vi "DAQ.vi"() -> ()   [LabVIEW 2018]
uses:
  <vilib>/userdefined/High Color/nirio_resource_hc.ctl
  Turbo Instrument Controller.llb/Type Def - Gauge Num Selection.ctl
  <vilib>/Utility/file.llb/Read Delimited Spreadsheet (DBL).vi
  <vilib>/FPGAPlugInAG/PXIe-7856R/niLvFpga_Open_PXIe-7856R.vi
  <vilib>/rvi/interface/nirviOpenFPGA/nirviOpenFPGA.xnode
  FPGA code/FPGA Bitfiles/Microspherefeedb_FPGATarget2_MultiChannelfFee_SMENcAWM-fA.lvbitx
  <instrlib>/Agilent 2000 3000 X-Series/Agilent 2000 3000 X-Series.lvlib
panel:
  in  "Synth_sync":bool
  in  "Scope only?":bool=TRUE
  in  "RIO Device":T1="RIO0"
  out "error out":errorcluster
  in  "Range (S)":dbl=0.002 format="%#_13g"
  in  "Use osciloscope chan 1":bool=TRUE
  in  "use single channel":bool
  in  "EOM":T2={"QWP"=FALSE, "QWP angles"="125,124,123,122,121,120,119,118,117,116,115,114,113,112,111,110,109,108,107,106,105,104,103,102,101,100,99,98,97,96,95,94,93,92,91,90,89,88,87,86,85,84,83,82,81,80,79,78,77,76,75,74,73,72,71,70,69,68,67,66,65,64,63,62,61,60,59,58,57,56,55,54,53,52,51,50,49,48,47,46,45,44,43,42,41,40,39,38,37,36,35,34,33,32,31,30,29,28,27,26,25,24,23,22,21", "reverse"=FALSE}
  out "Axes position":i32[](array[numeric])
  in  "Arb waveform path":path=path "C:/Users/UsphereLab/Documents/GitHub/Optlev/scripts/freq_comb/freq_comb_fixed4.txt"
  in  "Dipole average settings":T3={"Initial wait time"=5.0, "Number of steps"=10000, "CH1 Voltage"=13.5, "Use?"=FALSE, "CH2 Voltage"=13.5, "Variable Steps"=FALSE}
  in  "Stage settings":T4={"thetaY steps"=-12.0, "thetaZ steps"=-20.0, "Run thetaY?"=FALSE, "Run thetaZ?"=FALSE, "# repeats \n   in thetaY"=1, "# repeats \n   in thetaZ"=100}
  in  "Trigger Synth":bool
  in  "Enable Output?":bool
  out "P_cc [torr]":dbl format="%#_3g"
  out "P_pirani [torr]":dbl format="%#_3g"
  out "T_elec_rack [C]":dbl
  out "T_opt_table [C]":dbl
  in  "Read pressures?":bool
  in  "Flash lamp\n settings:":T5={"Flash lamp?"=FALSE, "Number of cyles\nbetween flashes"=1, "# Pulses"=1, "Stop flashing \nbelow thresh?"=FALSE, "Stop threshold"=0.02, "Pulse amp (V)"=0.001}
  in  "Synth settings:":T6={"start volt (V)"=0.0, "stop volt (V) "=0.0, "# V Steps"=1, "start freq (Hz)"=48.0, "stop freq (Hz) "=48.0, "# F steps"=1, "dc offset?"=FALSE, "start DC (V)"=0.0, "stop DC (V)"=0.0, "# DC steps "=1, "Set synth\n(HP33120A)?"=FALSE, "Use arbitrary\nwaveform?"=FALSE, "Arb waveform name:"="VOLATILE"}
  out "Waveform \nGraph":dbl[][](graph)
  out "Curr threshold":dbl
  in  "Number of Samples":dbl=100000.0
  in  "Sample Rate [Hz]":dbl=10000.0
  out "Actual Sample \nRate":dbl=10000.0 format="%0.2f"
  in  "Delay between files [s]":dbl caption="Delay Time (s)"
  in  "Num files":i32=1
  in  "File base name":string="rot9"
  in  "Directory path":path=path "C:/data/GADI"
  # "Logging Settings"
  # "How to use the channel/scope statements:\n\n\"use single channel\":\n\nis for measurement of rotation using the daq\nand high sample rate\n\n\n\n\"Scope only\" and  \"Use osciloscope chan 1\":\n\nonly uses the channel 1 of the scope\n\n\n\n \"Use osciloscope chan 1\":\n\nuses daq together with the channel 1 of the scope\n\nWarning: for this option to work, the number of samples per daq channel must be the same of the scope: ie; NS = 50e4"
  # "524288"
  # "Environment"
  # "Starts with the positive voltage\n\nIf Variable Steps is on, then the voltages in the synth's AC input and the voltages for the dipole will change for each step by 10% of the original voltage, so that we have voltages\n1*V volts, 0.9*V volts, 0.8*V volts, 0.7*V volts, and back again to V volts"
  # "Flash Lamp Settings"
  # "Acquired Data"
  # "Timing Settings"
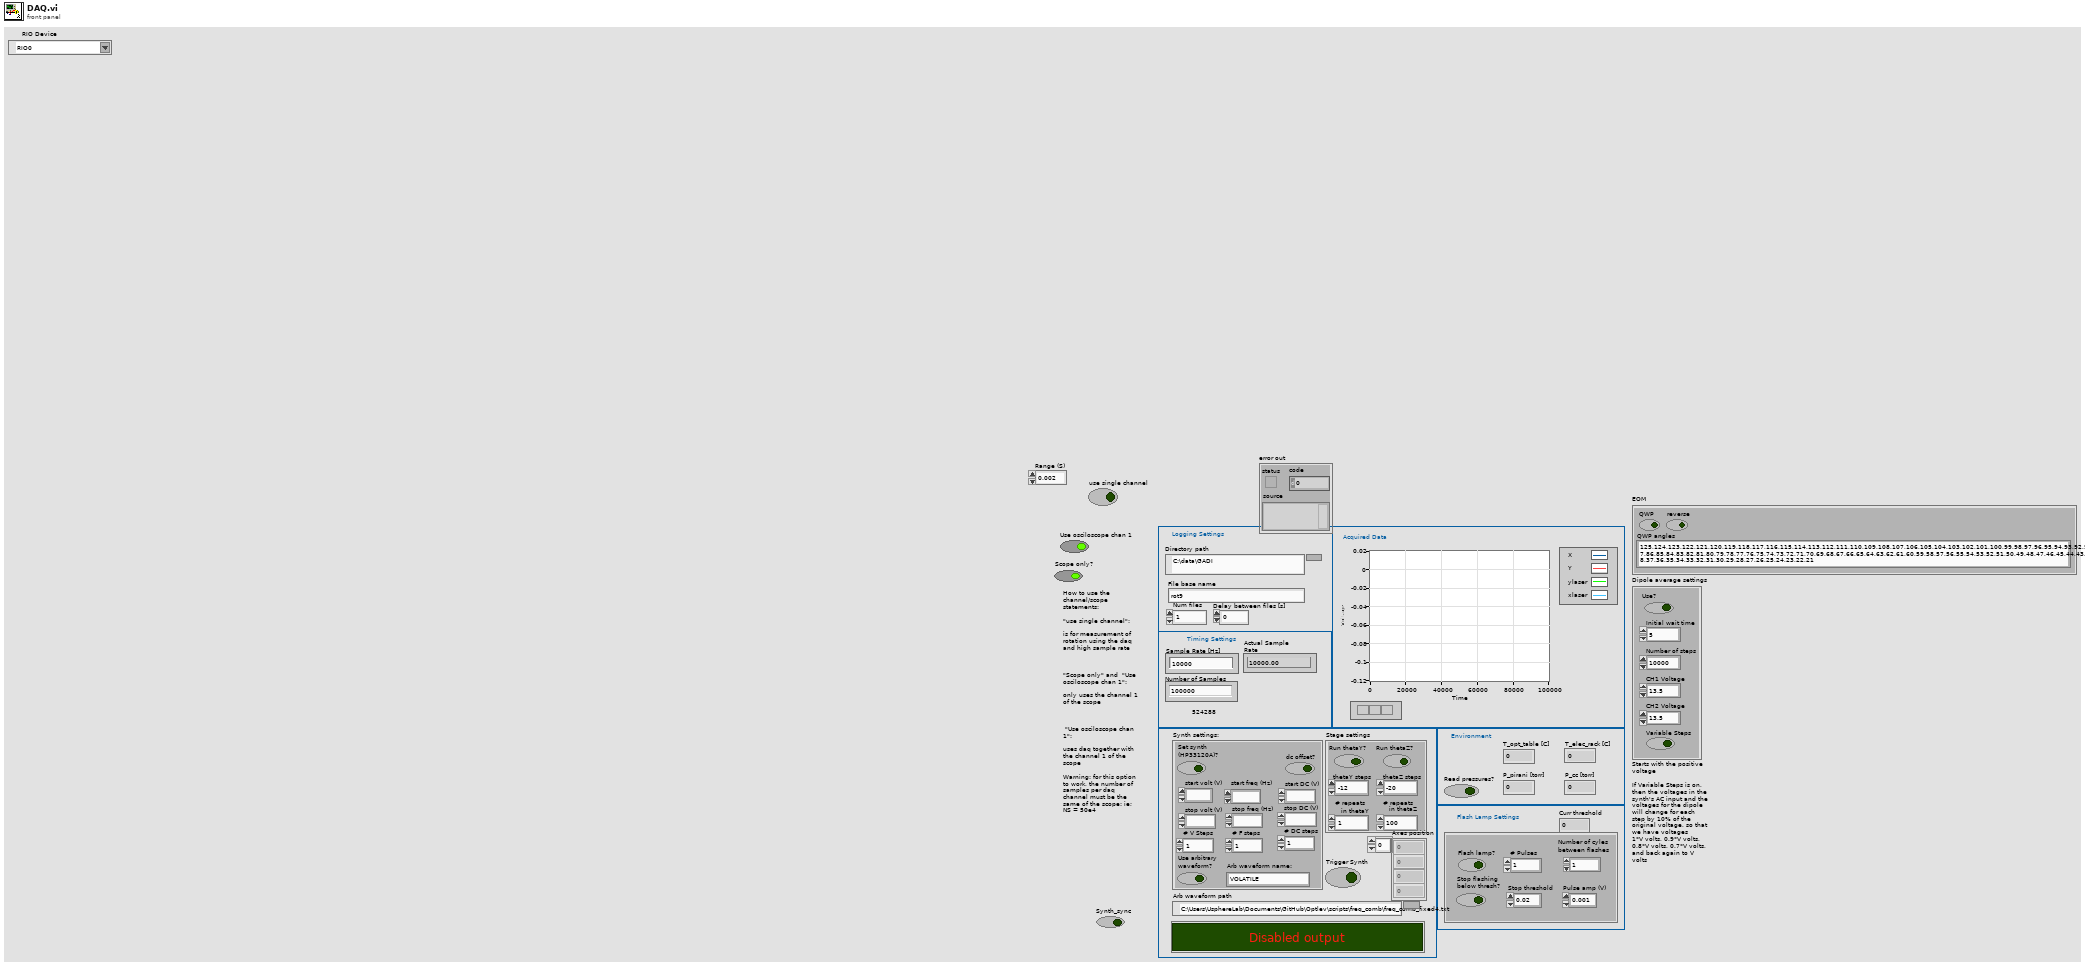
[diagram p1: front panel]
types:
  T1 = typedef "nirio_resource_hc.ctl" = tag
  T2 = cluster{"QWP":bool, "QWP angles":string, "reverse":bool}
  T3 = cluster{"Initial wait time":dbl, "Number of steps":i32, "CH1 Voltage":dbl, "Use?":bool, "CH2 Voltage":dbl, "Variable Steps":bool}
  T4 = cluster{"thetaY steps":dbl, "thetaZ steps":dbl, "Run thetaY?":bool, "Run thetaZ?":bool, "# repeats \n   in thetaY":i32, "# repeats \n   in thetaZ":i32}
  T5 = cluster{"Flash lamp?":bool, "Number of cyles\nbetween flashes":i32, "# Pulses":i32, "Stop flashing \nbelow thresh?":bool, "Stop threshold":dbl, "Pulse amp (V)":dbl}
  T6 = cluster{"start volt (V)":ext, "stop volt (V) ":ext, "# V Steps":i32, "start freq (Hz)":ext, "stop freq (Hz) ":ext, "# F steps":i32, "dc offset?":bool, "start DC (V)":ext, "stop DC (V)":ext, "# DC steps ":i32, "Set synth\n(HP33120A)?":bool, "Use arbitrary\nwaveform?":bool, "Arb waveform name:":string}
  T7 = cluster{"Tot Synth Arr":dbl[], "Tot Stage Arr":dbl[], "Stage Name Arr":dbl[], "QWP":dbl}[]
  T8 = cluster{"synth cluster":cluster{"VISA resource name out":refnum<visa-resource-name>, "error out":errorcluster}, "tilt stage config":cluster{"Y error out":errorcluster, "Y CmdLib Out":refnum<k24>, "Y Device Address":i32, "Y DeviceKey Out":string, "Z error out":errorcluster, "Z CmdLib Out":refnum<k24>, "Z Device Address":i32, "Z DeviceKey Out":string}}
  T9 = cluster{"Number of Samples":dbl, "Sample Rate [Hz]":dbl, "Physical Channels (Position signals)":tag, "Sample Clock Source":tag}
  T10 = typedef "Type Def - Gauge Num Selection.ctl" = enum16{"Gauge 1", "Gauge 2", "Gauge 3", "Gauge 4", "Gauge 5", "Gauge 6"}
  T11 = cluster{"Tot Synth Arr":dbl[], "Tot Stage Arr":dbl[], "Stage Name Arr":dbl[], "QWP":dbl}
  T12 = cluster{"Output channel (for flashing)":tag, i32, "path out":path, "Flash lamp\n settings:":cluster{"Flash lamp?":bool, "Number of cyles\nbetween flashes":i32, "# Pulses":i32, "Stop flashing \nbelow thresh?":bool, "Stop threshold":dbl, "Pulse amp (V)":dbl}}
  T13 = cluster{"Use arbitrary\nwaveform?":bool, "Arb waveform name:":string, "Enable Output?":bool, "Trigger Synth":bool, i32, "first row":dbl[]}
  T14 = cluster{"VISA resource name out":refnum<visa-resource-name>, "error out":errorcluster}
  T15 = cluster{"task out":refnum<k21>, "error out":errorcluster, "SampClk.Rate":dbl}
  T16 = cluster{"task out":refnum<k21>, "error out":errorcluster}
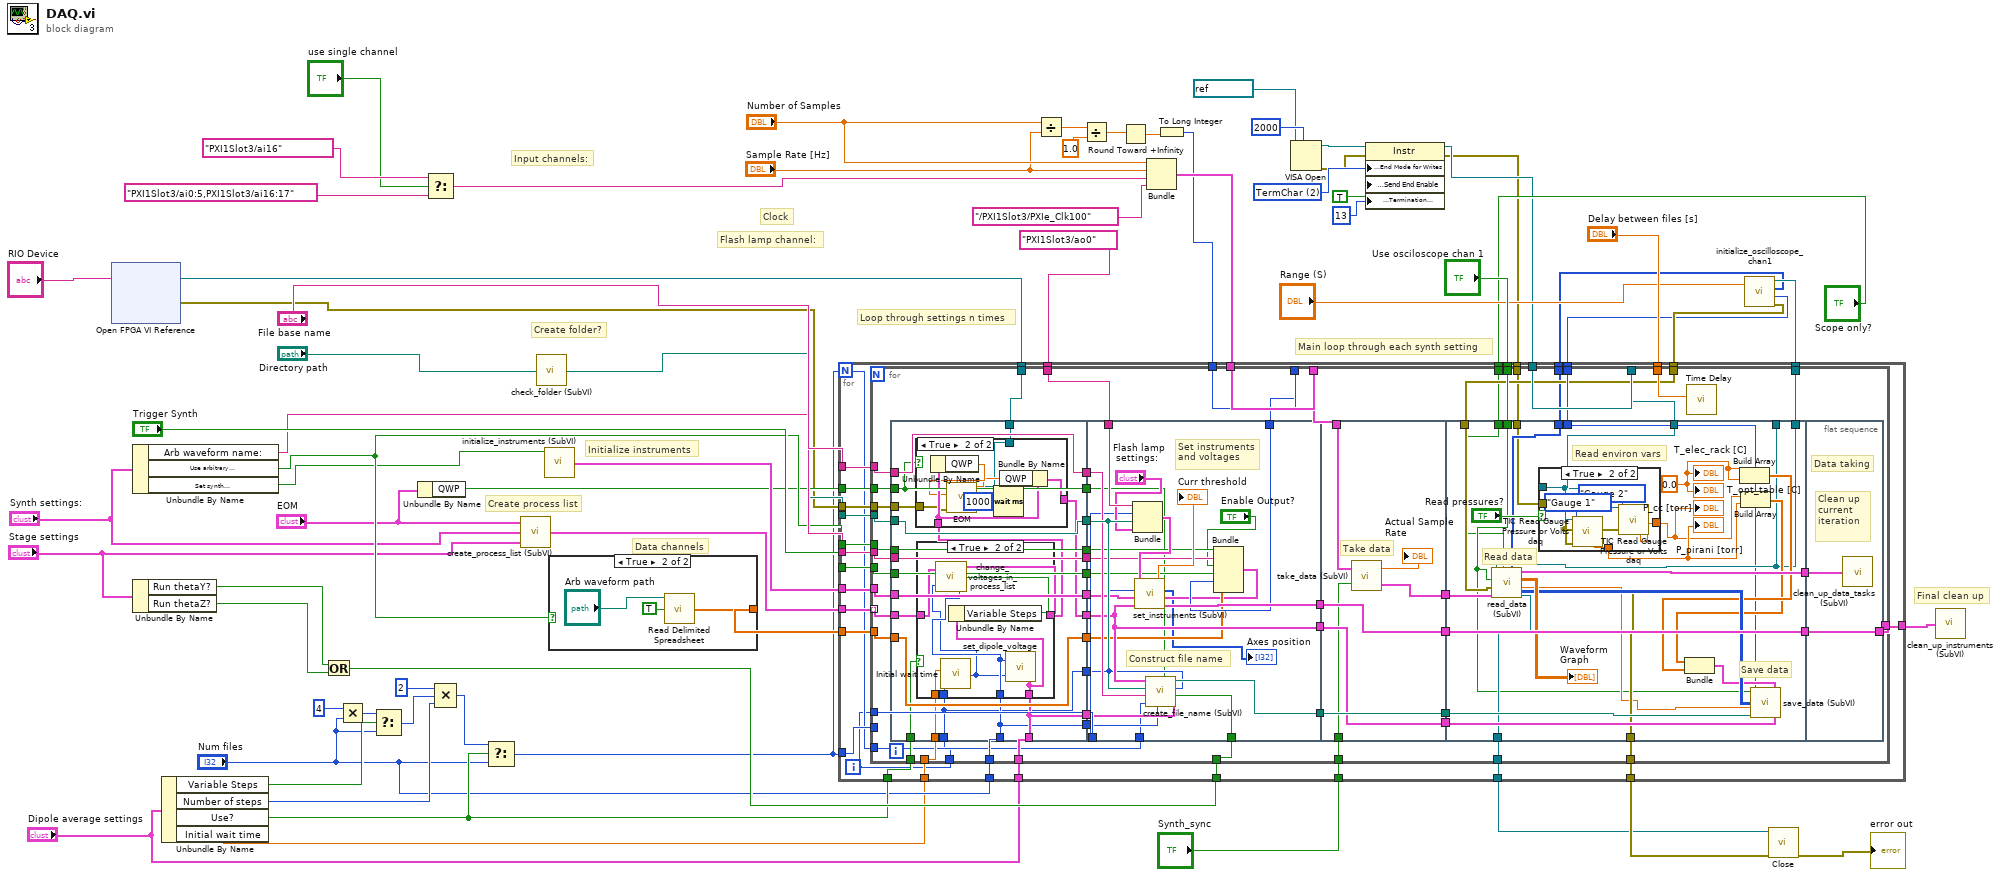
[diagram p0: block diagram]
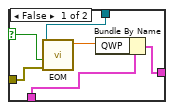
[diagram p2: hidden frame]
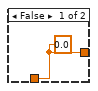
[diagram p4: hidden frame]
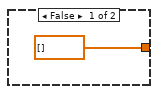
[diagram p5: hidden frame]
diagram:
  w8 = u16 2 items=["None", "Last Bit", "TermChar", "Break"] ("Serial Settings:End Mode for Writes")
  # "Main loop through each synth setting"
  # "Loop through settings n times"
  # "Final clean up"
  # "Initialize instruments"
  # "Create process list"
  # "Create folder?"
  # "Clock"
  # "Data channels"
  # "Flash lamp channel:"
  # "Input channels:"
  n1 = xnode "Open FPGA VI Reference"("resource name"="RIO Device") -> ("FPGA VI Reference Out"=w11:refnum<k20>, "error out"=w14:errorcluster)  [unwired: 1 in]
  n2 = Unbundle By Name("Synth settings:") -> ("Arb waveform name:"=w59:string, "Use arbitrary\nwaveform?"=w50:bool, "Set synth\n(HP33120A)?"=w43:bool)
  n3 = Unbundle By Name("Stage settings") -> ("Run thetaY?"=w48:bool, "Run thetaZ?"=w49:bool)
  n4 = Unbundle By Name("Dipole average settings") -> ("Variable Steps"=w37:bool, "Number of steps"=w41:i32, "Use?"=w38:bool, "Initial wait time"=w32:dbl)
  n5 = Or(x=w48, y=w49) -> (x .or. y?=w45:bool)
  n6 = Multiply(x=4, y="Num files") -> (x*y=w36:i32)
  n7 = Select(t=w36, s=w37, f="Num files") -> (s? t:f=w34:i32)
  n8 = Unbundle By Name("EOM") -> ("QWP"=w30:bool)
  n9 = Select(t=tag "PXI1Slot3/ai16" ("Physical Channels (Position signals)"), s="use single channel", f=tag "PXI1Slot3/ai0:5,PXI1Slot3/ai16:17" ("Physical Channels (Position signals)")) -> (s? t:f=w27:tag)
  n10 = Compound Arithmetic op=MULTIPLY(2 ("value"), w34, w41) -> (w40:i32)
  n11 = Select(t=w40, s=w38, f="Num files") -> (s? t:f=w12:i32)
  n12 = call "create_process_list (SubVI).vi"("Stage settings"="Stage settings", "Synth settings:"="Synth settings:", "Quarter Wave Plate"="EOM") -> ("Process list"=w55:T7)
  n13 = call "check_folder (SubVI).vi"("path in"="Directory path") -> ("path out"=w54:path)
  n14 = call "initialize_instruments (SubVI).vi"("Use synth?"=w43) -> ("initialized output"=w53:T8)  [unwired: 2 in]
  n15 = case shown="True" w50 {
    tunnel: [dbl[] [] ("first row") w72] -> w52
    frame False {
    }
    frame True {
      n16 = call-poly <vilib>:"Read Delimited Spreadsheet.vi"("file path (dialog if empty)"="Arb waveform path", "transpose? (F)"=TRUE) -> ("first row"=w72:dbl[])  [unwired: 8 in, 5 out]
    }
  }
  n17 = Divide(x="Number of Samples", y="Sample Rate [Hz]") -> (x/y=w63:dbl)
  n18 = Divide(x=w63, y=1.0) -> (x/y=w57:dbl)
  n19 = Round Toward +Infinity(x=w57) -> (ceil(x): smallest int >= x=w56:dbl)
  n20 = Bundle("Number of Samples"="Number of Samples", "Sample Rate [Hz]"="Sample Rate [Hz]", "Physical Channels (Position signals)"=w27, "Sample Clock Source"=tag "/PXI1Slot3/PXIe_Clk100") -> (w67:T9)  [unwired: 1 in]
  n21 = To Long Integer(number=w56) -> (32bit integer=w60:i32)
  n22 = VISA Open(timeout (0)=u32 2000 ("VISA Open timeout (0)"), VISA resource name=refnum<visa-resource-name> "COM7") -> (VISA resource name=w5:refnum<visa-resource-name>, error out=w4:errorcluster)  [unwired: 3 in]
  n23 = property class="Instr"(reference=w5, error in=w4, "Serial Settings:End Mode for Writes"=w8, "Message Based Settings:Send End Enable"=TRUE, "Message Based Settings:Termination Character"=u8 13) -> (reference out=w3:refnum<visa-resource-name>, error out=w1:errorcluster)
  n24 = call "initialize_oscilloscope_chan1.vi"("Range (0.001 S)"="Range (S)") -> ("VISA resource name out"=w18:refnum<visa-resource-name>, "channels"=w17:i32[], "number"=w16:i32, "error out"=w19:errorcluster)  [unwired: 1 in]
  n25 = for {
    N: w12 -> [w76]
    tunnel: w55 -> [w107]
    tunnel: tag "PXI1Slot3/ao0" ("Output channel (for flashing)") -> [w106]
    tunnel: w54 -> [w105]
    tunnel: w12 -> [w78]
    tunnel: "File base name" -> [w104]
    tunnel: w67 -> [w103]
    tunnel: [w102] -> w44
    tunnel: w50 -> [w101]
    tunnel: w59 -> [w100]
    tunnel: w3 -> [w99]
    tunnel: w60 -> [w98]
    tunnel: "Trigger Synth" -> [w97]
    tunnel: w52 -> [w96]
    tunnel: w45 -> [w95]
    tunnel: w53 -> [w94]
    tunnel: w32 -> [w93]
    tunnel: "Dipole average settings" -> [w92]
    tunnel: "Num files" -> [w91]
    tunnel: w38 -> [w90]
    tunnel: w30 -> [w89]
    tunnel: "Delay between files [s]" -> [w88]
    tunnel: "Use osciloscope chan 1" -> [w87]
    tunnel: w16 -> [w86]
    tunnel: [w85] -> w23
    tunnel: [w84] -> w22
    tunnel: w19 -> [w83]
    tunnel: w18 -> [w82]
    tunnel: w17 -> [w81]
    tunnel: w11 -> [w80]
    tunnel: w14 -> [w79]
    tunnel: "Scope only?" -> [w77]
    tunnel: "Synth_sync" -> [w74]
    tunnel: w1 -> [w73]
    i -> [w75]
    n26 = for {
      tunnel: w107 -> [w145] mode=indexing
      tunnel: w106 -> [w144]
      tunnel: w105 -> [w143]
      tunnel: w104 -> [w142]
      tunnel: w103 -> [w141]
      tunnel: [w140] -> w102
      tunnel: w101 -> [w139]
      tunnel: w100 -> [w138]
      tunnel: w99 -> [w137]
      tunnel: w98 -> [w136]
      tunnel: w97 -> [w135]
      tunnel: w96 -> [w134]
      tunnel: w95 -> [w133]
      tunnel: w94 -> [w132]
      tunnel: w93 -> [w131]
      tunnel: w92 -> [w130]
      tunnel: w91 -> [w129]
      tunnel: w90 -> [w128]
      tunnel: w75 -> [w127]
      tunnel: w78 -> [_]
      tunnel: w89 -> [w125]
      tunnel: w88 -> [w122]
      tunnel: w87 -> [w121]
      tunnel: w86 -> [w120]
      tunnel: [w119] -> w85
      tunnel: [w118] -> w84
      tunnel: w83 -> [w117]
      tunnel: w82 -> [w116]
      tunnel: w81 -> [w115]
      tunnel: w80 -> [w114]
      tunnel: w79 -> [w113]
      tunnel: w77 -> [w112]
      tunnel: w76 -> [w111]
      tunnel: w75 -> [w110]
      tunnel: w74 -> [w109]
      tunnel: w73 -> [w108]
      n27 = flat-sequence {
        tunnel: w132 -> [w175]
        tunnel: w134 -> [w176]
        tunnel: w135 -> [w177]
        tunnel: w138 -> [w178]
        tunnel: w139 -> [w179]
        tunnel: w142 -> [w180]
        tunnel: w143 -> [w181]
        tunnel: w145 -> [w169]
        tunnel: [w181] -> w163
        tunnel: [w180] -> w162
        tunnel: [w179] -> w161
        tunnel: [w178] -> w160
        tunnel: [w177] -> w159
        tunnel: [w176] -> w158
        tunnel: [w175] -> w157
        tunnel: w131 -> [w174]
        tunnel: w130 -> [w173]
        tunnel: [w173] -> w156
        tunnel: w129 -> [w171]
        tunnel: w128 -> [w172]
        tunnel: [w171] -> w155
        tunnel: w110 -> [w170]
        tunnel: [w170] -> w126
        tunnel: w125 -> [w168]
        tunnel: [w168] -> w124
        tunnel: [w166] -> w123
        tunnel: w114 -> [w165]
        tunnel: w113 -> [w164]
        tunnel: w144 -> [w227]
        tunnel: [w225] -> w154
        tunnel: [w222] -> w153
        tunnel: [w219] -> w152
        tunnel: w136 -> [w213]
        tunnel: w133 -> [w218]
        tunnel: w163 -> [w224]
        tunnel: w162 -> [w223]
        tunnel: w161 -> [w216]
        tunnel: w160 -> [w215]
        tunnel: w159 -> [w214]
        tunnel: w158 -> [w212]
        tunnel: w157 -> [w217]
        tunnel: w156 -> [w210]
        tunnel: w155 -> [w209]
        tunnel: w127 -> [w208]
        tunnel: w126 -> [w206]
        tunnel: w111 -> [w207]
        tunnel: w124 -> [w203]
        tunnel: w123 -> [w219]
        tunnel: [w229] -> w151
        tunnel: w154 -> [w229]
        tunnel: w141 -> [w233]
        tunnel: [w231] -> w150
        tunnel: [w232] -> w149
        tunnel: w153 -> [w232]
        tunnel: w152 -> [w230]
        tunnel: [w230] -> w148
        tunnel: w109 -> [w228]
        tunnel: [w259] -> w147
        tunnel: w151 -> [w259]
        tunnel: w150 -> [w258]
        tunnel: w149 -> [w255]
        tunnel: [w253] -> w146
        tunnel: w148 -> [w254]
        tunnel: w137 -> [w252]
        tunnel: w121 -> [w239]
        tunnel: w120 -> [w237]
        tunnel: [w245] -> w119
        tunnel: [w244] -> w118
        tunnel: [w242] -> _
        tunnel: w117 -> [w243]
        tunnel: w116 -> [w242]
        tunnel: w115 -> [w241]
        tunnel: w112 -> [w238]
        tunnel: w108 -> [w236]
        tunnel: w147 -> [w267]
        tunnel: w146 -> [w268]
        tunnel: [w267] -> w140
        frame #0 {
          n28 = case shown="True" w172 {
            tunnel: w174 -> [_ w202]
            tunnel: w173 -> [_ w198]
            tunnel: w171 -> [_ w197]
            tunnel: [w195 w201] -> w167
            tunnel: w169 -> [w195 w200]
            tunnel: w170 -> [_ w196]
            frame False {
            }
            frame True {
              n29 = call "Initial wait time"("Delay Time (s)"=w202) -> ()  [unwired: 10 in, 1 out]
              n30 = Unbundle By Name(w198) -> ("Variable Steps"=w199:bool)
              n31 = call "change_voltages_in_process_list.vi"("Process list"=w200, "iteration number"=w196, "Variable Steps"=w199, "Num files"=w197) -> ("output process list"=w201:T11)
              n32 = call "set_dipole_voltage.vi"("Dipole average settings"=w198, "iteration number"=w196, "Num files"=w197) -> ()
            }
          }
          n33 = case shown="True" w168 {
            selector: w168 -> [w186 _]
            tunnel: w167 -> [w184 w193]
            tunnel: [w183 w194] -> w166
            tunnel: w165 -> [w182 w188]
            tunnel: w164 -> [w187 w191]
            frame False {
              n34 = call "EOM.vi"("error in (no error)"=w187, "USE EOM?"=w186, "Refnum in"=w182) -> ("EOM_out"=w185:dbl)  [unwired: 8 in]
              n35 = Bundle By Name(cluster=w184, "QWP"=w185) -> (w183:T11)
            }
            frame True {
              n36 = Unbundle By Name(w193) -> ("QWP"=w190:dbl)
              n37 = call "EOM.vi"("error in (no error)"=w191, "EOM_amplitude"=w190, "Refnum in"=w188) -> ("EOM_out"=w189:dbl)  [unwired: 8 in]
              n38 = Wait (ms)(milliseconds to wait=u32 1000) -> ()  [unwired: 1 out]
              n39 = Bundle By Name(cluster=w193, "QWP"=w189) -> (w194:T11)
            }
          }
        }
        frame #1 {
          # "Construct file name"
          # "Set instruments and voltages"
          n40 = Bundle("Output channel (for flashing)"=w227, w208, "path out"=w224, "Flash lamp\n settings:"="Flash lamp\n settings:") -> (w220:T12)  [unwired: 1 in]
          n41 = call "create_file_name (SubVI).vi"("Dipole average settings"=w210, "stage on?"=w218, "file_idx"=w206, "QWP"=w203, "num files per step"=w209, "num files"=w207, "base name"=w223, "Path"=w224, "Process List"=w219) -> ("out path"=w222:path)
          n42 = Bundle("Use arbitrary\nwaveform?"=w216, "Arb waveform name:"=w215, "Enable Output?"="Enable Output?", "Trigger Synth"=w214, w213, "first row"=w212) -> (w211:T13)  [unwired: 1 in]
          n43 = call "set_instruments (SubVI).vi"("set_instrument inputs"=w211, "Process list"=w219, "initialized output"=w217, "flip iteration"=w206, "Flash lamp settings:"=w220) -> ("instrum out"=w225:T14, "Axes position"=→"Axes position":i32[], "Curr threshold"=→"Curr threshold":dbl)  [unwired: 1 in]
        }
        frame #2 {
          # "Take data"
          n44 = call "take_data (SubVI).vi"("Synth_sync"=w228, "channel settings"=w233) -> ("data tasks"=w231:T15, "Actual Sample Rate"=→"Actual Sample \nRate":dbl)
        }
        frame #3 {
          w246 = 0.0 ("T_elec_rack [C]")
          # "Read environ vars"
          # "Read data"
          # "Save data"
          n45 = call "read_data (SubVI).vi"("Channels"=w241, "Scope only?"=w238, "data tasks"=w258, "error in (no error)"=w243, "Use osciloscope chan 1"=w239, "VISA resource name"=w242) -> ("VISA resource name out"=w244:refnum<visa-resource-name>, "sample rate"=w240:dbl, "Output data"=→"Waveform \nGraph":dbl[][], "output data tasks"=w253:T16, "error out"=w245:errorcluster, "Rescaled data"=w256:i16[][])
          n46 = case shown="True" "Read pressures?" {
            tunnel: w252 -> [_ w266]
            tunnel: [w260 w262] -> w250
            tunnel: [w260 w261] -> w235
            tunnel: w236 -> [_ w265]
            frame False {
              w260 = 0.0 ("Scroll Pump Pressure 2 (mbar)")
            }
            frame True {
              n47 = call "TIC Read Gauge Pressure or Volts daq.vi"("VISA Session In"=w266, "Gauge Number (1)"=Type_Def_-_Gauge_Num_Selection."Gauge 1", "error in (no error)"=w265) -> ("mbar"=w262:dbl)  [unwired: 7 in, 5 out]
              n48 = call "TIC Read Gauge Pressure or Volts daq.vi"("VISA Session In"=w266, "Gauge Number (1)"=Type_Def_-_Gauge_Num_Selection."Gauge 2", "error in (no error)"=w265) -> ("mbar"=w261:dbl)  [unwired: 7 in, 5 out]
            }
          }
          "P_pirani [torr]" <- w250
          "P_cc [torr]" <- w235
          n49 = Build Array(w246, w246) -> (w248:dbl[])
          n50 = Build Array(w235, w250) -> (w247:dbl[])
          n51 = Bundle(w247, w248) -> (w249:cluster{dbl[], dbl[]})  [unwired: 1 in]
          n52 = call "save_data (SubVI).vi"("Scope True?"=w239, "Sample rate scope"=w237, "Sample rate"=w240, "Filename"=w255, "data"=w256, "environ cluster"=w249, "Process list"=w254) -> ()
          "T_opt_table [C]" <- w246
          "T_elec_rack [C]" <- w246
        }
        frame #4 {
          # "Data taking"
          # "Clean up\ncurrent iteration"
          n53 = call "clean_up_data_tasks (SubVI).vi"("data tasks"=w268) -> ()
        }
      }
      n54 = call "Time Delay"("Delay Time (s)"=w122) -> ()  [unwired: 10 in, 1 out]
    }
  }
  n55 = call <instrlib>:"Close.vi"("error in (no error)"=w23, "VISA resource name"=w22) -> ("error out"=→"error out":errorcluster)  [unwired: 9 in]
  n56 = call "clean_up_instruments (SubVI).vi"("instrum out"=w44) -> ()
